vi "Write Current Recipe Iterations.vi"(8 "error in (no error)":errorcluster, 10 "Current Recipe Iterations":dbl, 11 "Recipe State Data in":refnum<class "Recipe State Data.lvclass">) -> (0 "error out":errorcluster, 3 "Recipe State Data out":refnum<class "Recipe State Data.lvclass">)   [LabVIEW 2022 SP3, in "Recipe State Data.lvclass"]
uses:
  Recipe State Data.lvclass
  Recipe State Data.lvclass/Recipe State Data.ctl
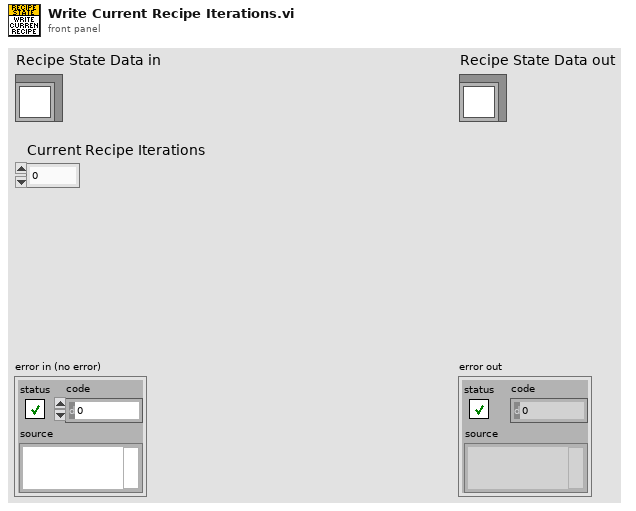
[diagram p1: front panel]
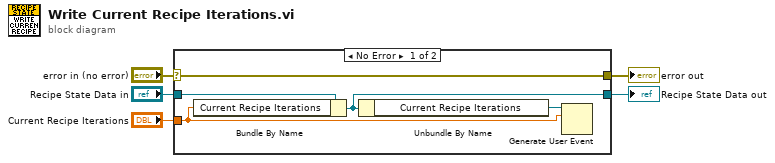
[diagram p0: block diagram]
diagram:
  n1 = case shown="No Error" "error in (no error)" {
    selector: "error in (no error)" -> [w10 w11]
    tunnel: [w10 w11] -> w4
    tunnel: [w8 w12] -> w2
    tunnel: "Recipe State Data in" -> [w9 w12]
    tunnel: "Current Recipe Iterations" -> [w6 _]
    frame No Error {
      n2 = Bundle By Name(cluster=w9, "Current Recipe Iterations"=w6) -> (w8:refnum<class "Recipe State Data.lvclass">)
      n3 = Unbundle By Name(w8) -> ("Current Recipe Iterations"=w7:refnum<user-event>)
      n4 = Generate User Event(user event=w7, event data cluster=w6) -> ()  [unwired: 2 in, 2 out]
    }
    frame Error {
    }
  }
  "error out" <- w4
  "Recipe State Data out" <- w2
